vi "Practica_4.vi"() -> ()   [LabVIEW 2020]
uses:
  <vilib>/express/express shared/transition.llb/Dynamic To Waveform Array.vi
  <vilib>/express/express signal manip/GetorSetDDTAttributes/Set DDT Attributes/SetT0.vi
  <vilib>/express/express shared/transition.llb/Waveform Array To Dynamic.vi
  <vilib>/express/express signal manip/GetorSetDDTAttributes/Set DDT Attributes/Set DDT Properties.xnode
panel:
  out "Waveform Chart":dynamicdata(graph)
  in  "stop":bool
  out "Máximo":dbl
  out "Mínimo":dbl
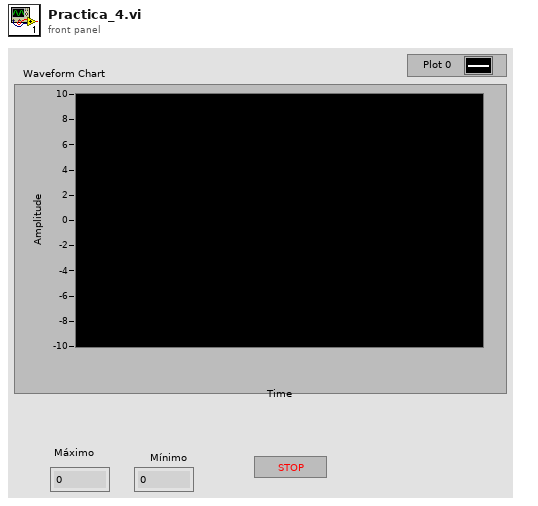
[diagram p1: front panel]
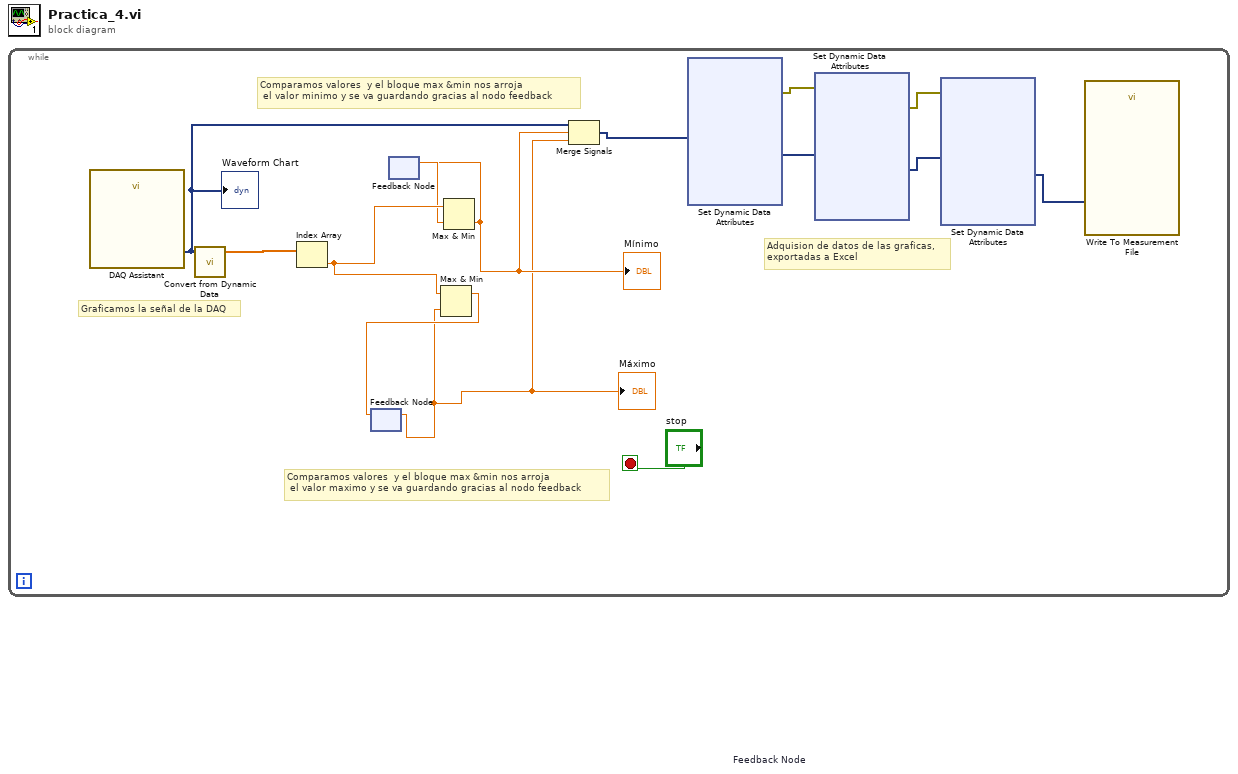
[diagram p0: block diagram]
diagram:
  n1 = while {
    stop <- "stop" stop-if-true
    # "Comparamos valores  y el bloque max &min nos arroja\n el valor maximo y se va guardando gracias al nodo feedback"
    # "Comparamos valores  y el bloque max &min nos arroja\n el valor minimo y se va guardando gracias al nodo feedback"
    # "Adquision de datos de las graficas,\nexportadas a Excel"
    # "Graficamos la señal de la DAQ"
    n2 = call "DAQ Assistant"() -> ("data"=w9:dynamicdata)  [unwired: 17 in, 2 out]
    "Waveform Chart" <- w9
    n3 = call "Convert from Dynamic Data"("Dynamic Data Type"=w9) -> ("Array"=w14:dbl[])  [unwired: 3 in]
    n4 = Index Array "Index Array"(array=w14) -> (element=w11:dbl)  [unwired: 1 in]
    n5 = feedback #1 "Feedback Node"() -> (w7:dbl)  [unwired: 1 in]
    "Máximo" <- w7
    n6 = feedback #2() -> (w10:dbl)  [unwired: 1 in]
    n7 = Max & Min(x=w11, y=w7) -> (max(x,y)=w12:dbl)  [unwired: 1 out]
    n8 = feedback-in #1(w12) -> ()
    n9 = Max & Min(x=w11, y=w10) -> (min(x,y)=w8:dbl)  [unwired: 1 out]
    "Mínimo" <- w8
    n10 = feedback-in #2(w8) -> ()
    n11 = Merge Signals "Merge Signals"(w9, w8, w7) -> (w6:dynamicdata)
    n12 = xnode "Set Dynamic Data Attributes"("Signals In"=w6) -> ("Signals Out"=w4:dynamicdata, "error out"=w5:errorcluster)  [unwired: 3 in]
    n13 = xnode "Set Dynamic Data Attributes"("Signals In"=w4, "error in"=w5) -> ("Signals Out"=w3:dynamicdata, "error out"=w2:errorcluster)  [unwired: 2 in]
    n14 = xnode "Set Dynamic Data Attributes"("Signals In"=w3, "error in"=w2) -> ("Signals Out"=w1:dynamicdata)  [unwired: 2 in, 1 out]
    n15 = call "Write To Measurement File"("Signals"=w1) -> ()  [unwired: 16 in, 3 out]
  }
